vi "OD-DarkBeforeEverySample.vi"() -> ()   [LabVIEW 2012]
uses:
  <vilib>/Instr/_visa.llb/VISA Find Search Mode.ctl
  <vilib>/Utility/file.llb/Write To Spreadsheet File (DBL).vi
  <vilib>/Utility/file.llb/Read From Spreadsheet File (string).vi
  <vilib>/Utility/file.llb/Write To Spreadsheet File (string).vi
  <userlib>/SPECcon/SPECcon.lvlib
panel:
  out "Samples Raw Data":dbl[][][](array[numeric])
  out "Dark 3":dbl[](array[numeric])
  out "Dark 2":dbl[](array[numeric])
  in  "Run Python Script\non 'log_OD.txt'":bool
  in  "from":i32=350
  in  "to":i32=1050
  in  "Automatic Measurement":bool
  in  "Interval in minutes":dbl
  out "Absorbance [AU] vs. Wavelength [nm]":cluster{dbl[], dbl[]}[](graph)
  out "Reference":dbl[](array[numeric])
  out "Number of bytes read":i32
  out "Raw Data":string
  out "Command sent":string
  in  "Integration Time":i32=100
  in  "Average":i32=10
  out "info return":i32
  out "info out":string
  out "Connected?":bool
  out "Identified?":bool
  out "firmware out":string
  out "Port":string caption="element"
  in  "index":i32
  in  "Connect to this port?":bool caption="Connect to this port"
  in  "Reset the graph for\nnext run":bool
  # "Connection"
  # "Data Acquisition"
  # "Measurement Settings"
  # "Wavelength Range (nm)"
  # "-"
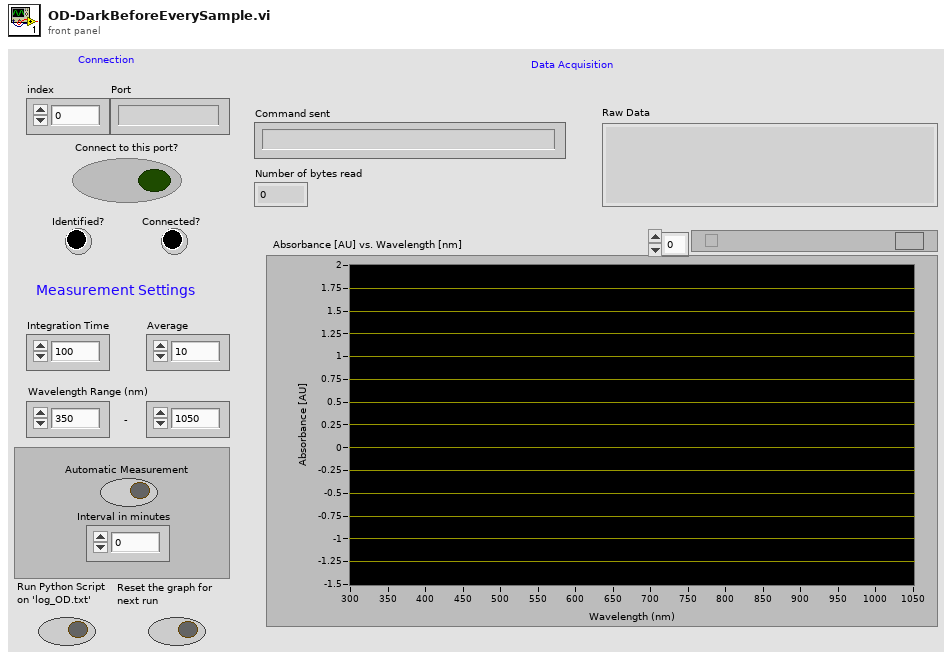
[diagram p1: front panel]
types:
  T1 = typedef "VISA Find Search Mode.ctl" = u32
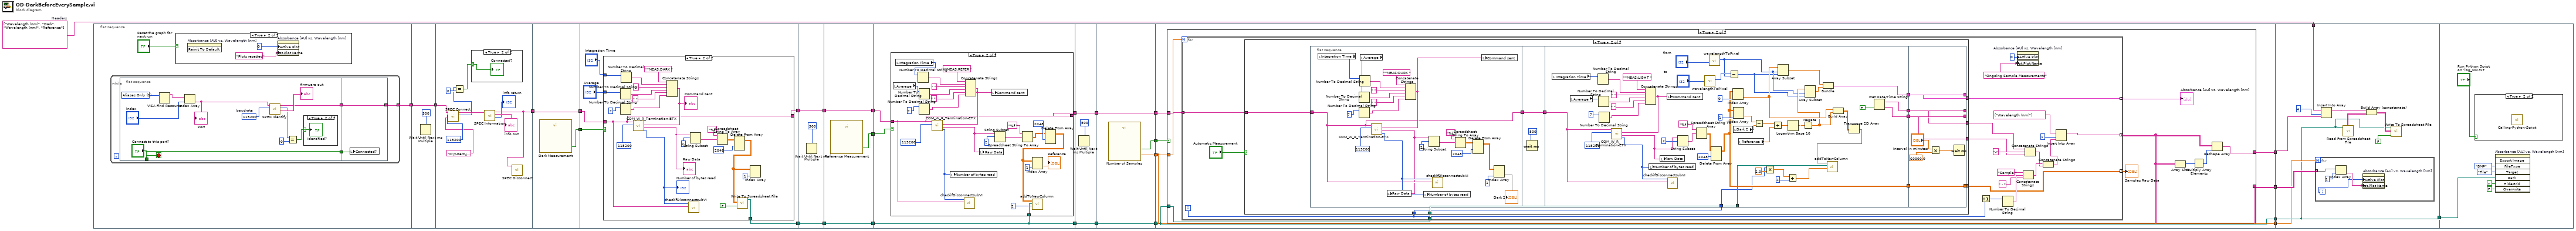
[diagram p0: block diagram]
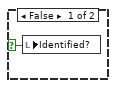
[diagram p3: hidden frame]
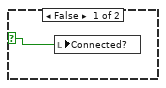
[diagram p4: hidden frame]
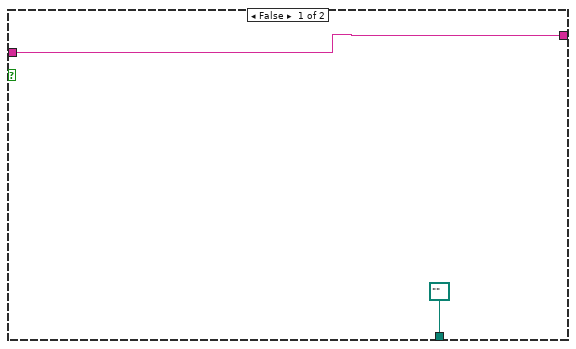
[diagram p5: hidden frame]
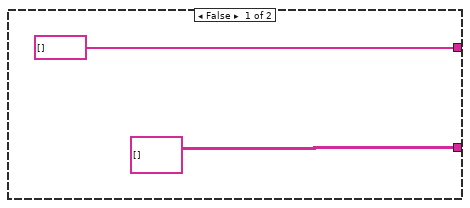
[diagram p7: hidden frame]
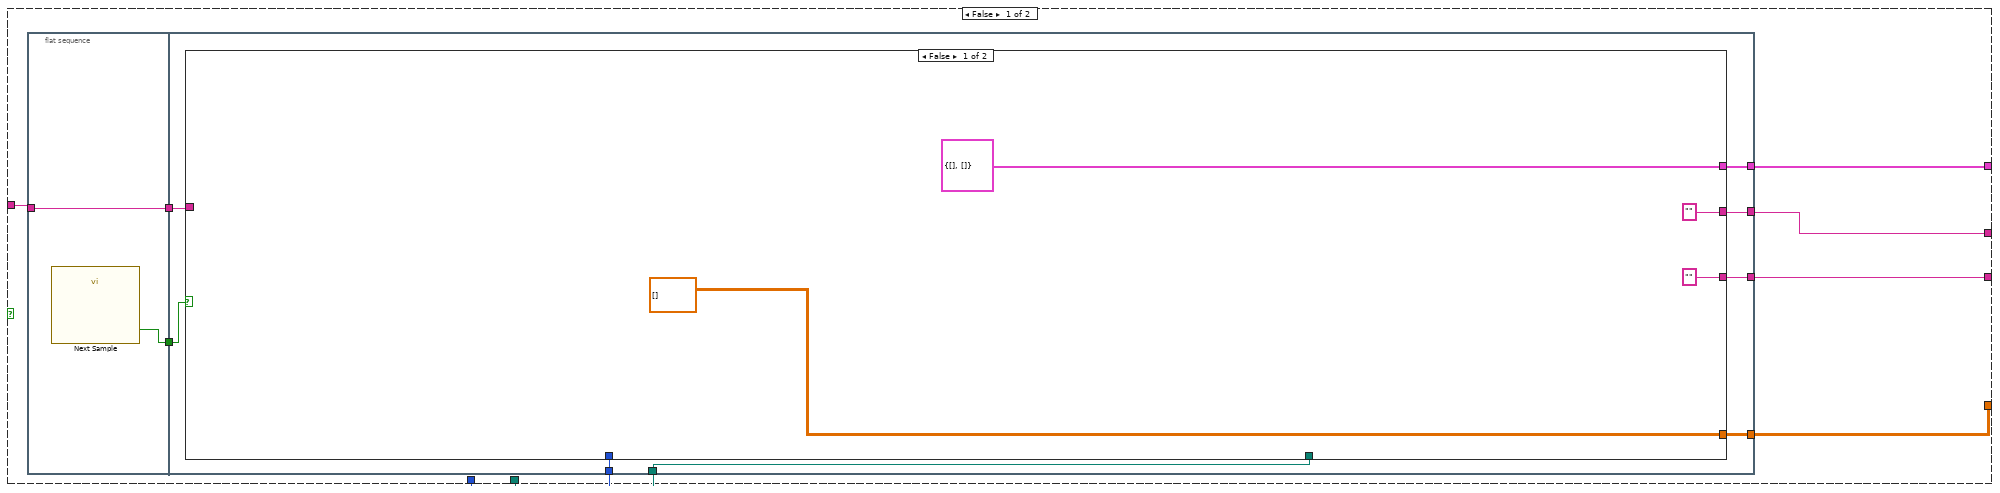
[diagram p8: hidden frame]
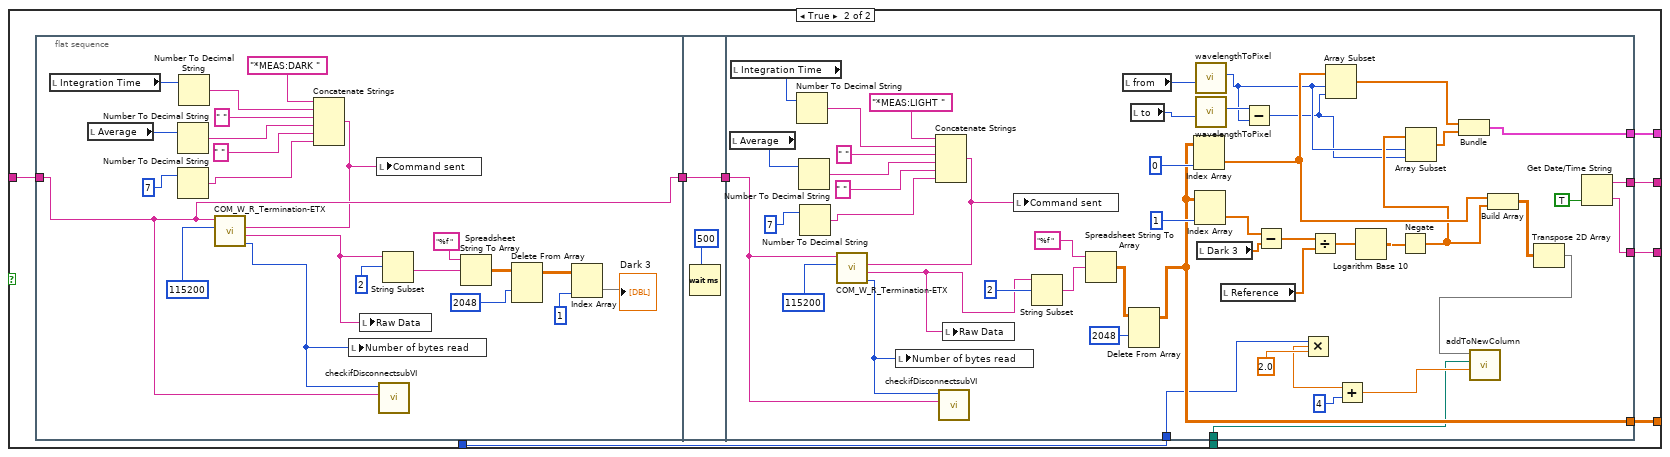
[diagram p9: hidden frame]
diagram:
  w2 = string[] ["Wavelength (nm)", "Dark", "Wavelength (nm)", "Reference"]  # Headers
  n1 = flat-sequence {
    tunnel: [w28] -> w26
    tunnel: w26 -> [w50]
    tunnel: [w50] -> w25
    tunnel: w25 -> [w58]
    tunnel: [w55] -> w24
    tunnel: [w65] -> w23
    tunnel: w24 -> [w65]
    tunnel: [w64] -> w22
    tunnel: w23 -> [w70]
    tunnel: w22 -> [w71]
    tunnel: [w66] -> w21
    tunnel: [w67] -> w20
    tunnel: [w98] -> w19
    tunnel: w21 -> [w98]
    tunnel: [w97] -> w18
    tunnel: w20 -> [w97]
    tunnel: [w102] -> w17
    tunnel: w19 -> [w102]
    tunnel: [w101] -> w16
    tunnel: [w100] -> w15
    tunnel: w18 -> [w100]
    tunnel: w17 -> [w106]
    tunnel: w16 -> [w105]
    tunnel: [w104] -> w14
    tunnel: [w103] -> w13
    tunnel: w15 -> [w103]
    tunnel: [w133] -> w12
    tunnel: w14 -> [w133]
    tunnel: [w132] -> w11
    tunnel: w13 -> [w132]
    tunnel: [w138] -> w10
    tunnel: [w137] -> w9
    tunnel: [w136] -> w8
    tunnel: w12 -> [w136]
    tunnel: [w135] -> w7
    tunnel: w11 -> [w135]
    tunnel: w10 -> [w144]
    tunnel: w9 -> [w141]
    tunnel: w8 -> [w143]
    tunnel: w7 -> [w139]
    tunnel: [w142] -> w6
    tunnel: [w141] -> w5
    tunnel: [w140] -> w4
    tunnel: [w139] -> w1
    tunnel: w2 -> [w384]
    tunnel: w6 -> [w382]
    tunnel: w5 -> [w376]
    tunnel: w4 -> [w377]
    tunnel: [w375] -> w3
    tunnel: w1 -> [w375]
    tunnel: w3 -> [w389]
    frame #0 {
      n2 = while {
        tunnel: [w34] -> w28
        stop <- w33 stop-if-true
        n3 = flat-sequence {
          tunnel: ["Connect to this port?"] -> w33
          tunnel: [w40] -> w32
          tunnel: ["Connect to this port?"] -> w31
          tunnel: [w49] -> w34
          tunnel: w32 -> [w49]
          tunnel: w31 -> [w48]
          frame #0 {
            w42 = T1 2 items=["Canonical Names Only"=0, "Aliases Only"=2, "Include Matching Aliases"=3, "Include All Aliases"=4] ("Search Mode")
            w45 = 115200  # baudrate
            n4 = VISA Find Resource(10:w42) -> (3:w41:string[])  [unwired: 2 in, 2 out]
            n5 = Index Array(array=w41, index="index") -> (element=w39:string)
            "Port" <- w39
            n6 = call <userlib>:"SPEC Identify.vi"("baudrate_or_mode"=w45, "port_number"=w39) -> ("firmware out"=→"firmware out":string, "function return"=w38:i32, "port_number out"=w40:string)  [unwired: 7 in]
            n7 = Equal?(x=w38, y=0) -> (x = y?=w36:bool)
            n8 = case shown="True" w36 {
              selector: w36 -> [w46 w47]
              frame False {
                n9 = local write "Identified?"(w46) -> ()
              }
              frame True {
                "Identified?" <- w47
              }
            }
          }
          frame #1 {
            n10 = local write "Connected?"(w48) -> ()
          }
        }
      }
      n11 = case shown="True" "Reset the graph for\nnext run" {
        frame False {
        }
        frame True {
          n12 = invoke on="Absorbance [AU] vs. Wavelength [nm]" class="XYGraph (strict)" method="Reinit To Default"() -> ()  [unwired: 3 in, 3 out]
          n13 = property on="Absorbance [AU] vs. Wavelength [nm]" class="XYGraph (strict)"("Active Plot"=u32 0, "Plot.Plot Name"="Plots resetted") -> ()  [unwired: 2 in, 2 out]
        }
      }
    }
    frame #1 {
      n14 = Wait Until Next ms Multiple(millisecond multiple=u32 500) -> ()  [unwired: 1 out]
    }
    frame #2 {
      n15 = call <userlib>:"SPEC Connect.vi"("filename"="C:\\Users\\Frederic Schmitt\\Desktop\\GE\\Optical Density - Sinan\\SPECview\\SPECcon_1.3\\example_CS.txt", "baudrate"=115200, "port_number"=w58) -> ("function return"=w52:i32, "port_number out"=w59:string)  [unwired: 6 in, 1 out]
      n16 = Equal?(x=w52, y=0) -> (x = y?=w53:bool)
      n17 = case shown="True" w53 {
        selector: w53 -> [w62 w63]
        frame False {
          n18 = local write "Connected?"(w62) -> ()
        }
        frame True {
          "Connected?" <- w63
        }
      }
      n19 = call <userlib>:"SPEC Information.vi"("port_number"=w59) -> ("function return"=→"info return":i32, "info out"=→"info out":string, "port_number out"=w55:string)  [unwired: 8 in]
      n20 = call <userlib>:"SPEC Disconnect.vi"("port_number"=w55) -> ()  [unwired: 9 in, 2 out]
    }
    frame #3 {
      n21 = call "Dark Measurement"() -> ("Sure"=w64:bool)  [unwired: 18 in, 1 out]
    }
    frame #4 {
      n22 = case shown="True" w71 {
        tunnel: w70 -> [w73 w74]
        tunnel: [w73 w74] -> w66
        tunnel: "Integration Time" -> [_ w88]
        tunnel: "Average" -> [_ w87]
        tunnel: [path "" ("new file path (Not A Path if cancelled)") w81] -> w67
        frame False {
        }
        frame True {
          n23 = Number To Decimal String(number=w87) -> (decimal integer string=w92:string)  [unwired: 1 in]
          n24 = Number To Decimal String(number=7) -> (decimal integer string=w90:string)  [unwired: 1 in]
          n25 = Number To Decimal String(number=w88) -> (decimal integer string=w94:string)  [unwired: 1 in]
          n26 = Concatenate Strings("*MEAS:DARK ", w94, " ", w92, " ", w90) -> (w78:string)
          "Command sent" <- w78
          n27 = call "COM_W_R_Termination-ETX.vi"("VISA resource name"=w74, "baud rate"=u32 115200, "string to write"=w78) -> ("read string"=w85:string, "return count"=w77:u32)  [unwired: 6 in]
          "Number of bytes read" <- w77
          "Raw Data" <- w85
          n28 = call "checkifDisconnectsubVI.vi"("port_number in"=w74, "function return 3"=w77) -> ()  [unwired: 10 in]
          n29 = String Subset(string=w85, offset (0)=2 ("offset")) -> (substring=w83:string)  [unwired: 1 in]
          n30 = Spreadsheet String To Array(format string="%f ", spreadsheet string=w83) -> (array=w79:dbl[][])  [unwired: 2 in]
          n31 = Delete From Array(array=w79, index (row)=2048) -> (array with subset deleted=w75:dbl[][])  [unwired: 2 in, 1 out]
          n32 = call-poly <vilib>:"Write To Spreadsheet File.vi"("append to file? (new file:F)"=FALSE, "2D data"=w75) -> ("new file path (Not A Path if cancelled)"=w81:path)  [unwired: 6 in]
          n33 = Index Array(array=w75, index (col)=1 ("disabled index (col)")) -> ()  [unwired: 1 in, 1 out]
        }
      }
    }
    frame #5 {
      n34 = Wait Until Next ms Multiple(millisecond multiple=u32 500) -> ()  [unwired: 1 out]
    }
    frame #6 {
      n35 = call "Reference Measurement"() -> ("Sure"=w101:bool)  [unwired: 18 in, 1 out]
    }
    frame #7 {
      n36 = case shown="True" w105 {
        tunnel: w106 -> [w107 w108]
        tunnel: [w107 w108] -> w104
        tunnel: w103 -> [_ w118]
        frame False {
        }
        frame True {
          n37 = local read "Average"() -> (w123:i32)
          n38 = local read "Integration Time"() -> (w122:i32)
          n39 = Number To Decimal String(number=w122) -> (decimal integer string=w129:string)  [unwired: 1 in]
          n40 = Number To Decimal String(number=w123) -> (decimal integer string=w127:string)  [unwired: 1 in]
          n41 = Number To Decimal String(number=7) -> (decimal integer string=w125:string)  [unwired: 1 in]
          n42 = Concatenate Strings("*MEAS:REFER ", w129, " ", w127, " ", w125) -> (w114:string)
          n43 = call "COM_W_R_Termination-ETX.vi"("VISA resource name"=w108, "baud rate"=u32 115200, "string to write"=w114) -> ("read string"=w113:string, "return count"=w112:u32)  [unwired: 6 in]
          n44 = local write "Number of bytes read"(w112) -> ()
          n45 = call "checkifDisconnectsubVI.vi"("port_number in"=w108, "function return 3"=w112) -> ()  [unwired: 10 in]
          n46 = local write "Raw Data"(w113) -> ()
          n47 = local write "Command sent"(w114) -> ()
          n48 = String Subset(string=w113, offset (0)=2 ("offset")) -> (substring=w119:string)  [unwired: 1 in]
          n49 = Spreadsheet String To Array(format string="%f ", spreadsheet string=w119) -> (array=w115:dbl[][])  [unwired: 2 in]
          n50 = Delete From Array(array=w115, index (row)=2048) -> (array with subset deleted=w111:dbl[][])  [unwired: 2 in, 1 out]
          n51 = Index Array(array=w111, index (col)=1 ("disabled index (col)")) -> (element=→"Reference":dbl[])  [unwired: 1 in]
          n52 = call "addToNewColumn.vi"("disabled index (col)"=2, "new file path (Not A Path if cancelled)"=w118, "Array"=w111) -> ()  [unwired: 9 in]
        }
      }
    }
    frame #8 {
      n53 = Wait Until Next ms Multiple(millisecond multiple=u32 500) -> ()  [unwired: 1 out]
    }
    frame #9 {
      n54 = call "Number of Samples"() -> ("number_samples"=w137:dbl, "OK"=w138:bool)  [unwired: 17 in, 1 out]
    }
    frame #10 {
      n55 = case shown="True" w144 {
        tunnel: w141 -> [_ w154]
        tunnel: w143 -> [_ w155]
        tunnel: w139 -> [_ w147]
        tunnel: [string[] [] w152] -> w142
        tunnel: [string[][] [] ("array") w149] -> w140
        frame False {
        }
        frame True {
          n56 = for {
            N: w154 -> [_]
            tunnel: w155 -> [w176]
            tunnel: [w156] -> w148 mode=indexing
            tunnel: w147 -> [w175]
            tunnel: [w170] -> w149 mode=indexing
            tunnel: [w164] -> w150 mode=indexing
            i -> [w161]
            n57 = case shown="True" "Automatic Measurement" {
              tunnel: w176 -> [w183 w294]
              tunnel: [w182 w293] -> w156
              tunnel: w175 -> [w181 w290]
              tunnel: w161 -> [w177 w289]
              tunnel: [w180 w286] -> w164
              tunnel: [w178 w287] -> w158
              tunnel: [w179 w288] -> w157
              frame False {
                n58 = flat-sequence {
                  tunnel: w183 -> [w187]
                  tunnel: [w187] -> w185
                  tunnel: [w186] -> w184
                  tunnel: w185 -> [w195]
                  tunnel: w184 -> [w194]
                  tunnel: [w193] -> w182
                  tunnel: w177 -> [w192]
                  tunnel: w181 -> [w188]
                  tunnel: [w191] -> w180
                  tunnel: [w190] -> w179
                  tunnel: [w189] -> w178
                  frame #0 {
                    n59 = call "Next Sample"() -> ("OK"=w186:bool)  [unwired: 18 in, 1 out]
                  }
                  frame #1 {
                    n60 = case shown="False" w194 {
                      tunnel: w195 -> [_ w208]
                      tunnel: [dbl[][] [] w207] -> w193
                      tunnel: w192 -> [_ w200]
                      tunnel: [cluster{dbl[], dbl[]} {[], []} w206] -> w191
                      tunnel: ["" ("time string") w205] -> w190
                      tunnel: ["" ("date string") w204] -> w189
                      tunnel: w188 -> [_ w201]
                      frame False {
                      }
                      frame True {
                        n61 = flat-sequence {
                          tunnel: w208 -> [w215]
                          tunnel: [w215] -> w203
                          tunnel: w203 -> [w232]
                          tunnel: [w232] -> w202
                          tunnel: [w253] -> w207
                          tunnel: w200 -> [w234]
                          tunnel: w201 -> [w233]
                          tunnel: [w249] -> w206
                          tunnel: w202 -> [w240]
                          tunnel: [w244] -> w205
                          tunnel: [w243] -> w204
                          frame #0 {
                            n62 = local read "Integration Time"() -> (w213:i32)
                            n63 = local read "Average"() -> (w212:i32)
                            n64 = Number To Decimal String(number=w212) -> (decimal integer string=w226:string)  [unwired: 1 in]
                            n65 = Number To Decimal String(number=7) -> (decimal integer string=w224:string)  [unwired: 1 in]
                            n66 = Number To Decimal String(number=w213) -> (decimal integer string=w228:string)  [unwired: 1 in]
                            n67 = Concatenate Strings("*MEAS:DARK ", w228, " ", w226, " ", w224) -> (w214:string)
                            n68 = call "COM_W_R_Termination-ETX.vi"("VISA resource name"=w215, "baud rate"=u32 115200, "string to write"=w214) -> ("read string"=w209:string, "return count"=w211:u32)  [unwired: 6 in]
                            n69 = local write "Number of bytes read"(w211) -> ()
                            n70 = local write "Raw Data"(w209) -> ()
                            n71 = local write "Command sent"(w214) -> ()
                            n72 = call "checkifDisconnectsubVI.vi"("port_number in"=w215, "function return 3"=w211) -> ()  [unwired: 10 in]
                            n73 = String Subset(string=w209, offset (0)=2 ("offset")) -> (substring=w220:string)  [unwired: 1 in]
                            n74 = Spreadsheet String To Array(format string="%f ", spreadsheet string=w220) -> (array=w218:dbl[][])  [unwired: 2 in]
                            n75 = Delete From Array(array=w218, index (row)=2048) -> (array with subset deleted=w216:dbl[][])  [unwired: 2 in, 1 out]
                            n76 = Index Array(array=w216, index (col)=1 ("disabled index (col)")) -> (element=→"Dark 3":dbl[])  [unwired: 1 in]
                          }
                          frame #1 {
                            n77 = Wait (ms)(milliseconds to wait=u32 500) -> ()  [unwired: 1 out]
                          }
                          frame #2 {
                            n78 = local read "Average"() -> (w251:i32)
                            n79 = local read "Integration Time"() -> (w250:i32)
                            n80 = Number To Decimal String(number=w250) -> (decimal integer string=w279:string)  [unwired: 1 in]
                            n81 = Number To Decimal String(number=w251) -> (decimal integer string=w277:string)  [unwired: 1 in]
                            n82 = Number To Decimal String(number=7) -> (decimal integer string=w275:string)  [unwired: 1 in]
                            n83 = Concatenate Strings("*MEAS:LIGHT ", w279, " ", w277, " ", w275) -> (w248:string)
                            n84 = call "COM_W_R_Termination-ETX.vi"("VISA resource name"=w240, "baud rate"=u32 115200, "string to write"=w248) -> ("read string"=w247:string, "return count"=w241:u32)  [unwired: 6 in]
                            n85 = local write "Number of bytes read"(w241) -> ()
                            n86 = call "checkifDisconnectsubVI.vi"("port_number in"=w240, "function return 3"=w241) -> ()  [unwired: 10 in]
                            n87 = local write "Raw Data"(w247) -> ()
                            n88 = local write "Command sent"(w248) -> ()
                            n89 = String Subset(string=w247, offset (0)=2 ("offset")) -> (substring=w271:string)  [unwired: 1 in]
                            n90 = Spreadsheet String To Array(format string="%f ", spreadsheet string=w271) -> (array=w254:dbl[][])  [unwired: 2 in]
                            n91 = local read "from"() -> (w239:i32)
                            n92 = Delete From Array(array=w254, index (row)=2048) -> (array with subset deleted=w253:dbl[][])  [unwired: 2 in, 1 out]
                            n93 = local read "to"() -> (w238:i32)
                            n94 = Index Array(array=w253, index (col)=0 ("disabled index (col)")) -> (element=w258:dbl[])  [unwired: 1 in]
                            n95 = Index Array(array=w253, index (col)=1 ("disabled index (col)")) -> (element=w269:dbl[])  [unwired: 1 in]
                            n96 = call "wavelengthToPixel.vi"("w"=w239) -> ("r1"=w236:i32)  [unwired: 8 in, 1 out]
                            n97 = call "wavelengthToPixel.vi"("w"=w238) -> ("r1"=w237:i32)  [unwired: 8 in, 1 out]
                            n98 = local read "Dark 3"() -> (w242:dbl[])
                            n99 = local read "Reference"() -> (w246:dbl[])
                            n100 = Subtract(x=w237, y=w236) -> (x-y=w235:i32)
                            n101 = Subtract(x=w269, y=w242) -> (x-y=w268:dbl[])
                            n102 = Multiply(x=w234, y=2.0) -> (x*y=w259:dbl)
                            n103 = Divide(x=w268, y=w246) -> (x/y=w267:dbl[])
                            n104 = Array Subset(array=w258, index=w236, length=w235) -> (w257:dbl[])
                            n105 = Add(x=w259, y=4) -> (x+y=w263:dbl)
                            n106 = Logarithm Base 10(1:w267) -> (0:w266:dbl[])
                            n107 = Negate(x=w266) -> (-x=w256:dbl[])
                            n108 = Array Subset(array=w256, index=w236, length=w235) -> (w255:dbl[])
                            n109 = Bundle(w257, w255) -> (w249:cluster{dbl[], dbl[]})  [unwired: 1 in]
                            n110 = Build Array(w258, w256) -> (w262:dbl[][])
                            n111 = Transpose 2D Array(2D array=w262) -> (transposed array=w261:dbl[][])
                            n112 = call "addToNewColumn.vi"("disabled index (col)"=w263, "new file path (Not A Path if cancelled)"=w233, "Array"=w261) -> ()  [unwired: 9 in]
                            n113 = Get Date/Time String(want seconds? (F)=TRUE) -> (date string=w243:string, time string=w244:string)  [unwired: 2 in]
                          }
                        }
                      }
                    }
                  }
                }
              }
              frame True {
                n114 = flat-sequence {
                  tunnel: w294 -> [w296]
                  tunnel: [w296] -> w291
                  tunnel: [w318] -> w292
                  tunnel: w291 -> [w318]
                  tunnel: w290 -> [w367]
                  tunnel: w289 -> [w319]
                  tunnel: w292 -> [w320]
                  tunnel: [w324] -> w285
                  tunnel: [w321] -> w284
                  tunnel: [w322] -> w283
                  tunnel: [w323] -> w282
                  tunnel: [w371] -> w288
                  tunnel: [w372] -> w287
                  tunnel: [w373] -> w286
                  tunnel: [w374] -> w293
                  tunnel: w285 -> [w374]
                  tunnel: w284 -> [w373]
                  tunnel: w283 -> [w372]
                  tunnel: w282 -> [w371]
                  frame #0 {
                    n115 = local read "Integration Time"() -> (w298:i32)
                    n116 = Number To Decimal String(number=7) -> (decimal integer string=w309:string)  [unwired: 1 in]
                    n117 = Number To Decimal String(number=w298) -> (decimal integer string=w313:string)  [unwired: 1 in]
                    n118 = local read "Average"() -> (w316:i32)
                    n119 = Number To Decimal String(number=w316) -> (decimal integer string=w311:string)  [unwired: 1 in]
                    n120 = Concatenate Strings("*MEAS:DARK ", w313, " ", w311, " ", w309) -> (w300:string)
                    n121 = call "COM_W_R_Termination-ETX.vi"("VISA resource name"=w296, "baud rate"=u32 115200, "string to write"=w300) -> ("read string"=w295:string, "return count"=w299:u32)  [unwired: 6 in]
                    n122 = local write "Raw Data"(w295) -> ()
                    n123 = local write "Number of bytes read"(w299) -> ()
                    n124 = String Subset(string=w295, offset (0)=2 ("offset")) -> (substring=w305:string)  [unwired: 1 in]
                    n125 = call "checkifDisconnectsubVI.vi"("port_number in"=w296, "function return 3"=w299) -> ()  [unwired: 10 in]
                    n126 = Spreadsheet String To Array(format string="%f ", spreadsheet string=w305) -> (array=w303:dbl[][])  [unwired: 2 in]
                    n127 = Delete From Array(array=w303, index (row)=2048) -> (array with subset deleted=w297:dbl[][])  [unwired: 2 in, 1 out]
                    n128 = local write "Command sent"(w300) -> ()
                    n129 = Index Array(array=w297, index (col)=1 ("disabled index (col)")) -> (element=→"Dark 2":dbl[])  [unwired: 1 in]
                  }
                  frame #1 {
                    n130 = Wait (ms)(milliseconds to wait=u32 500) -> ()  [unwired: 1 out]
                  }
                  frame #2 {
                    n131 = local read "Integration Time"() -> (w358:i32)
                    n132 = local read "Average"() -> (w357:i32)
                    n133 = Number To Decimal String(number=w358) -> (decimal integer string=w364:string)  [unwired: 1 in]
                    n134 = Number To Decimal String(number=w357) -> (decimal integer string=w362:string)  [unwired: 1 in]
                    n135 = Number To Decimal String(number=7) -> (decimal integer string=w360:string)  [unwired: 1 in]
                    n136 = Concatenate Strings("*MEAS:LIGHT ", w364, " ", w362, " ", w360) -> (w330:string)
                    n137 = call "COM_W_R_Termination-ETX.vi"("VISA resource name"=w320, "baud rate"=u32 115200, "string to write"=w330) -> ("read string"=w329:string, "return count"=w325:u32)  [unwired: 6 in]
                    n138 = local write "Number of bytes read"(w325) -> ()
                    n139 = local write "Raw Data"(w329) -> ()
                    n140 = local write "Command sent"(w330) -> ()
                    n141 = call "checkifDisconnectsubVI.vi"("port_number in"=w320, "function return 3"=w325) -> ()  [unwired: 10 in]
                    n142 = String Subset(string=w329, offset (0)=2 ("offset")) -> (substring=w354:string)  [unwired: 1 in]
                    n143 = Spreadsheet String To Array(format string="%f ", spreadsheet string=w354) -> (array=w337:dbl[][])  [unwired: 2 in]
                    n144 = call "wavelengthToPixel.vi"("w"="to") -> ("r1"=w333:i32)  [unwired: 8 in, 1 out]
                    n145 = call "wavelengthToPixel.vi"("w"="from") -> ("r1"=w332:i32)  [unwired: 8 in, 1 out]
                    n146 = Delete From Array(array=w337, index (row)=2048) -> (array with subset deleted=w324:dbl[][])  [unwired: 2 in, 1 out]
                    n147 = Subtract(x=w333, y=w332) -> (x-y=w331:i32)
                    n148 = Index Array(array=w324, index (col)=0 ("disabled index (col)")) -> (element=w341:dbl[])  [unwired: 1 in]
                    n149 = Index Array(array=w324, index (col)=1 ("disabled index (col)")) -> (element=w352:dbl[])  [unwired: 1 in]
                    n150 = local read "Dark 2"() -> (w326:dbl[])
                    n151 = local read "Reference"() -> (w328:dbl[])
                    n152 = Subtract(x=w352, y=w326) -> (x-y=w351:dbl[])
                    n153 = Multiply(x=w319, y=2.0) -> (x*y=w342:dbl)
                    n154 = Divide(x=w351, y=w328) -> (x/y=w350:dbl[])
                    n155 = Array Subset(array=w341, index=w332, length=w331) -> (w340:dbl[])
                    n156 = Add(x=w342, y=4) -> (x+y=w346:dbl)
                    n157 = Logarithm Base 10(1:w350) -> (0:w349:dbl[])
                    n158 = Negate(x=w349) -> (-x=w339:dbl[])
                    n159 = Array Subset(array=w339, index=w332, length=w331) -> (w338:dbl[])
                    n160 = Bundle(w340, w338) -> (w321:cluster{dbl[], dbl[]})  [unwired: 1 in]
                    n161 = Build Array(w341, w339) -> (w345:dbl[][])
                    n162 = Transpose 2D Array(2D array=w345) -> (transposed array=w344:dbl[][])
                    n163 = call "addToNewColumn.vi"("disabled index (col)"=w346, "new file path (Not A Path if cancelled)"=w367, "Array"=w344) -> ()  [unwired: 9 in]
                    n164 = Get Date/Time String(want seconds? (F)=TRUE) -> (date string=w322:string, time string=w323:string)  [unwired: 2 in]
                  }
                  frame #3 {
                    n165 = Multiply(x="Interval in minutes", y=60000.0 ("x")) -> (x*y=w370:dbl)
                    n166 = Wait (ms)(milliseconds to wait=w370) -> ()  [unwired: 1 out]
                  }
                }
              }
            }
            n167 = Increment(x=w161) -> (x+1=w163:i32)
            n168 = Number To Decimal String(number=w163) -> (decimal integer string=w169:string)  [unwired: 1 in]
            n169 = property on="Absorbance [AU] vs. Wavelength [nm]" class="XYGraph (strict)"("Active Plot"=u32 0, "Plot.Plot Name"="Ongoing Sample Measurements") -> ()  [unwired: 2 in, 2 out]
            n170 = Concatenate Strings("Sample ", w169, " - " ("string")) -> (w166:string)
            n171 = Concatenate Strings(w158, "-" ("string"), w157) -> (w165:string)
            n172 = Concatenate Strings(w166, w165) -> (w162:string)
            n173 = Insert Into Array(array=string[] ["Wavelength (nm)"], index=1, new element=w162) -> (w170:string[])
          }
          "Absorbance [AU] vs. Wavelength [nm]" <- w150
          "Samples Raw Data" <- w148
          n174 = Array Size(array=w149) -> (size(s)=w151:i32[])
          n175 = Multiply Array Elements(1:w151) -> (0:w153:i32)
          n176 = Reshape Array(w149, w153) -> (w152:string[])
        }
      }
    }
    frame #11 {
      n177 = for {
        N: w376 -> [_]
        tunnel: w377 -> [w388] mode=indexing
        i -> [w385]
        n178 = Index Array(array=w388, index=1) -> (element=w386:string)
        n179 = property on="Absorbance [AU] vs. Wavelength [nm]" class="XYGraph (strict)"("Active Plot"=w385, "Plot.Plot Name"=w386) -> ()  [unwired: 2 in, 2 out]
      }
      n180 = Insert Into Array(array=w384, index=4, new element=w382) -> (w381:string[])
      n181 = call-poly <vilib>:"Read From Spreadsheet File.vi"("file path (dialog if empty)"=w375) -> ("all rows"=w380:string[][])  [unwired: 6 in, 4 out]
      n182 = Build Array (concatenate)(w381, w380) -> (w379:string[][])
      n183 = call-poly <vilib>:"Write To Spreadsheet File.vi"("append to file? (new file:F)"=FALSE, "2D data"=w379, "file path (dialog if empty)"=w375) -> ()  [unwired: 5 in, 1 out]
    }
    frame #12 {
      n184 = case shown="True" "Run Python Script\non 'log_OD.txt'" {
        frame False {
        }
        frame True {
          n185 = call "Calling-Python-Script.vi"() -> ()  [unwired: 1 in]
        }
      }
      n186 = invoke on="Absorbance [AU] vs. Wavelength [nm]" class="XYGraph (strict)" method="Export Image"("FileType"=enum32{"BMP", "EPS", "EMF", "PICT"}."BMP" ("File Type"), "Target"=enum32{"File", "Clipboard"}."File", "Path"=w389, "HideGrid"=TRUE ("Hide Grid"), "Overwrite"=FALSE ("Always Overwrite")) -> ()  [unwired: 3 in, 8 out]
    }
  }
